vi "CHR 63205 ELoad.vi"   [LabVIEW 2018]
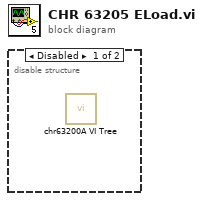
[diagram p0: block diagram]
diagram:
  n1 = disable-structure shown="Disabled" {
    frame Disabled {
      n2 = call <instrlib>:"chr63200A VI Tree.vi"() -> ()  [unwired: 12 in]
    }
    frame Enabled {
    }
  }
